vi "Pockels Cal-Obtain power meter scaling.vi"() -> (3 "Power meter scaling/cal":string[][](array[string])=[["mW", "mV"], ["0", "0"], ["21", "139"], ["43", "285"], ["65", "433"], ["88", "579"], ["109", "726"], ["130", "868"], ["152", "1009"], ["173", "1155"], ["192", "1280"], ["205", "1370"]])   [LabVIEW 2017]
uses:
  Typedefs/Which path.ctl
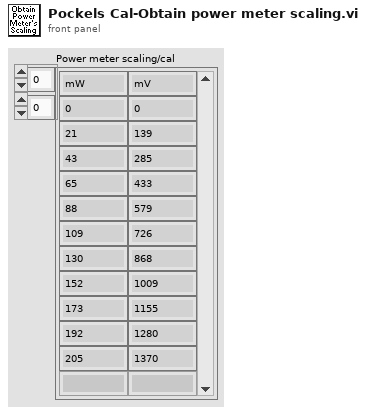
[diagram p1: front panel]
types:
  T1 = typedef "Which path.ctl" = enum16{"Configuration Files", "Calibration Files", "Images", "Setup.ini", "Loaded User profile.ini", "User's-Previous session.ini", "New user profile.ini", "Selected User profile.ini", "User profiles folder", "Power meter scaling.txt", "FOV Cal.ini"}
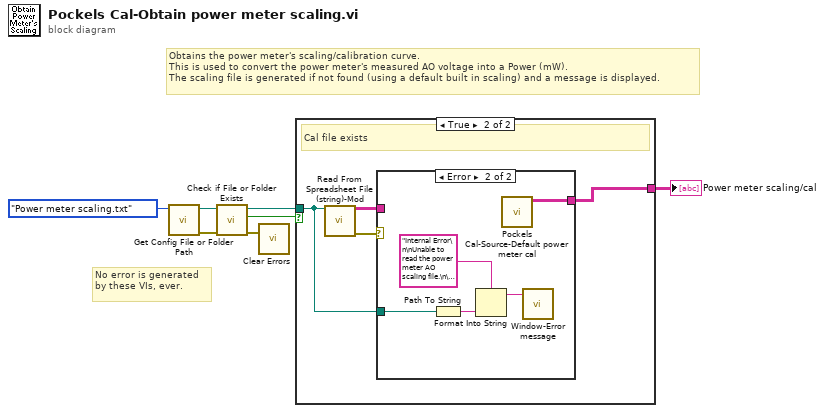
[diagram p0: block diagram]
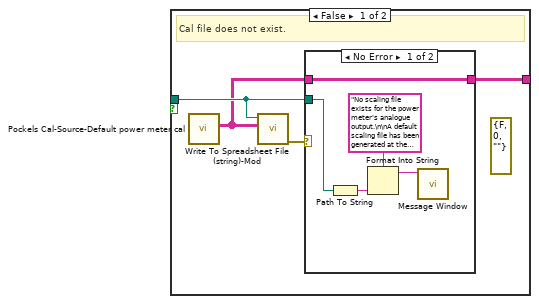
[diagram p2: hidden frame]
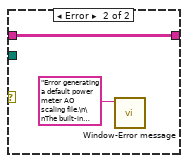
[diagram p3: hidden frame]
diagram:
  # "Obtains the power meter's scaling/calibration curve.\nThis is used to convert the power meter's measured AO voltage into a Power (mW).\nThe scaling file is generated if not found (using a default built in scaling) and a message is displayed."
  # "No error is generated by these VIs, ever."
  n1 = call "Get Config File or Folder Path.vi"("Which file or folder?"=Which_path."Power meter scaling.txt") -> ("Error Out"=w6:errorcluster, "File Path"=w3:path)  [unwired: 8 in, 1 out]
  n2 = call <vilib>:"Check if File or Folder Exists.vi"("error in (no error)"=w6, "path"=w3) -> ("error out"=w7:errorcluster, "file or folder exists?"=w4:bool, "dup path"=w5:path)  [unwired: 7 in]
  n3 = call <vilib>:"Clear Errors.vi"("error in (no error)"=w7) -> ()  [unwired: 5 in, 2 out]
  n4 = case shown="True" w4 {
    tunnel: [w8 w20] -> w1
    tunnel: w5 -> [w11 w19]
    frame False {
      (unwired) errorcluster {"status"=FALSE, "code"=0, "source"=""} ("error IO")
      # "Cal file does not exist."
      n5 = call "Pockels Cal-Source-Default power meter cal.vi"() -> ("Default power meter cal"=w9:string[][])  [unwired: 11 in]
      n6 = call <userlib>:"Write To Spreadsheet File (string)-Mod.vi"("2D data"=w9, "file path (dialog if empty)"=w11) -> ("error out"=w10:errorcluster)  [unwired: 8 in, 1 out]
      n7 = case shown="No Error" w10 {
        tunnel: w11 -> [w14 _]
        tunnel: w9 -> [w13 w18]
        tunnel: [w13 w18] -> w8
        frame No Error {
          n8 = Path To String(path=w14) -> (string=w16:string)
          n9 = Format Into String(format string="No scaling file exists for the power meter's analogue output.\n\nA default scaling file has been generated at the path shown below. The default scaling is valid for the Coherent FieldMate power meter when it is set to its \">3\" setting with no decimal point.\n\nIf you are not using a Coherent FieldMate for the automatic Pockels calibration, please open the file manually in Excel and update it with valid values ensuring that it contains at least two measurements.\n\nThe first column is the power displayed on the meter. The second column is the power meter's output voltage corresponding to each measured power. \n\nYou should disable auto-ranging on the meter and set it to an optimal measurement range to maximise measurement accuracy.\n\nNote that the first pair of values should be always zero.\n\nFile Path:\n%s\n" ("Message"), w16) -> (resulting string=w15:string)  [unwired: 2 in, 1 out]
          n10 = call "Message Window.vi"("Message string"=w15) -> ()  [unwired: 10 in, 1 out]
        }
        frame Error {
          n11 = call "Window-Error message.vi"("Message"="Error generating a default power meter AO scaling file.\n\nThe built-in default power meter scaling has been used.") -> ()  [unwired: 10 in, 1 out]
        }
      }
    }
    frame True {
      # "Cal file exists"
      n12 = call <userlib>:"Read From Spreadsheet File (string)-Mod.vi"("file path (dialog if empty)"=w19) -> ("all rows"=w21:string[][], "error out"=w22:errorcluster)  [unwired: 9 in, 4 out]
      n13 = case shown="Error" w22 {
        tunnel: w21 -> [w23 _]
        tunnel: [w23 w28] -> w20
        tunnel: w19 -> [_ w25]
        frame No Error {
        }
        frame Error {
          n14 = Path To String(path=w25) -> (string=w26:string)
          n15 = Format Into String(format string="Internal Error\n\nUnable to read the power meter AO scaling file.\n\nThe built-in default power meter scaling has been used.\n\nFile path:\n%s" ("Message"), w26) -> (resulting string=w27:string)  [unwired: 2 in, 1 out]
          n16 = call "Pockels Cal-Source-Default power meter cal.vi"() -> ("Default power meter cal"=w28:string[][])  [unwired: 11 in]
          n17 = call "Window-Error message.vi"("Message"=w27) -> ()  [unwired: 10 in, 1 out]
        }
      }
    }
  }
  "Power meter scaling/cal" <- w1
